vi "String History Cacher.vi"(7 "length":i32=10000, 10 "Include Timestamp(F)":bool, 11 "String":string) -> (3 "String Cache":string)   [LabVIEW 2014]
doc: "Return the <b>String Cache</b> containing <b>length</b> number of characters, including the new input <b>String</b>."
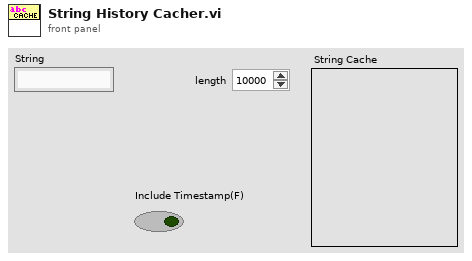
[diagram p1: front panel]
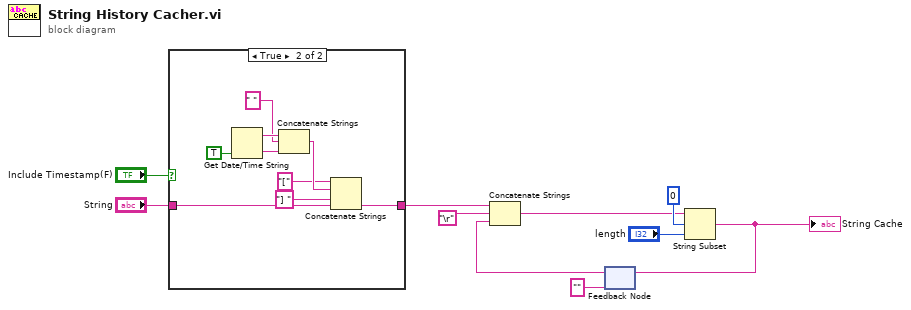
[diagram p0: block diagram]
diagram:
  n1 = case shown="True" "Include Timestamp(F)" {
    tunnel: "String" -> [w11 w20]
    tunnel: [w11 w16] -> w2
    frame False {
    }
    frame True {
      n2 = Get Date/Time String(want seconds? (F)=TRUE) -> (date string=w18:string, time string=w17:string)  [unwired: 2 in]
      n3 = Concatenate Strings(w18, " " ("string"), w17) -> (w15:string)
      n4 = Concatenate Strings("[" ("string"), w15, "] " ("string"), w20) -> (w16:string)
    }
  }
  n5 = feedback #1("") -> (w5:string)
  n6 = Concatenate Strings(w2, "\r", w5) -> (w4:string)
  n7 = String Subset(string=w4, offset (0)=0, length (rest)="length") -> (substring=w3:string)
  "String Cache" <- w3
  n8 = feedback-in #1(w3) -> ()
